vi "DB -Path.vi"() -> (3 "String":string)   [LabVIEW 2015]
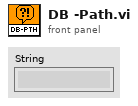
[diagram p1: front panel]
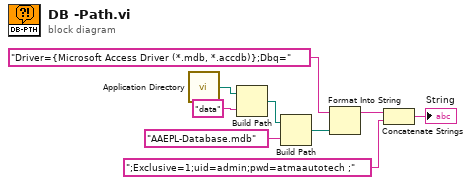
[diagram p0: block diagram]
diagram:
  n1 = call <vilib>:"Application Directory.vi"() -> ("Application Directory"=w1:path)
  n2 = Build Path(base path=w1, name or relative path="data") -> (appended path=w2:path)
  n3 = Build Path(base path=w2, name or relative path="AAEPL-Database.mdb") -> (appended path=w3:path)
  n4 = Format Into String(initial string="Driver={Microsoft Access Driver (*.mdb, *.accdb)};Dbq=" ("name or relative path"), w3) -> (resulting string=w7:string)  [unwired: 2 in, 1 out]
  n5 = Concatenate Strings(w7, ";Exclusive=1;uid=admin;pwd=atmaautotech ;") -> (→"String":string)
